vi "CDMA_TxSpreading.vi"(5 "ch_sf_tx":dbl, 7 "ch_code_tx":dbl, 8 "error in (no error)":errorcluster caption="错误输入（无错误）", 9 "input_dataq":dbl[](array[numeric]), 10 "input_datai":dbl[](array[numeric]), 11 "Path":path) -> (0 "error out":errorcluster caption="错误输出", 2 "sf_data":cdb[](array[numeric]), 3 "Path Out":path)   [LabVIEW 2015]
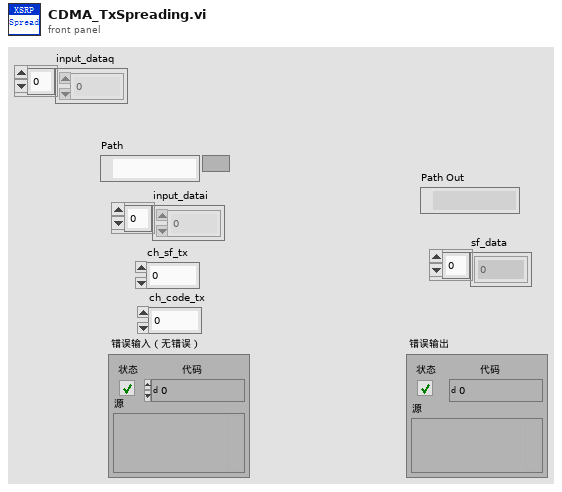
[diagram p1: front panel]
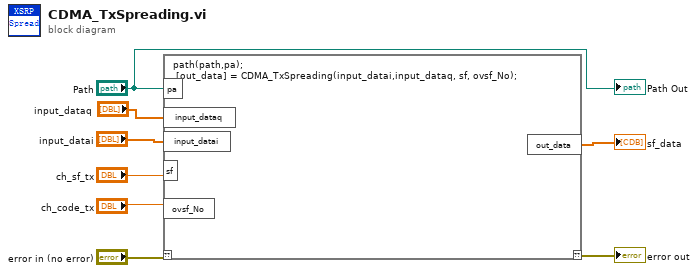
[diagram p0: block diagram]
diagram:
  n1 = script code="path(path,pa);\n [out_data] = CDMA_TxSpreading(input_datai,input_dataq, sf, ovsf_No);"("??"="error in (no error)", "pa"="Path", "input_datai"="input_datai", "sf"="ch_sf_tx", "ovsf_No"="ch_code_tx", "input_dataq"="input_dataq") -> ("??"=→"error out":errorcluster, "out_data"=→"sf_data":cdb[])
  "Path Out" <- "Path"
